vi "Drive Mode.vi"   [LabVIEW 2016]
uses:
  <vilib>/Rock Robotics/WPI/Camera/WPI_CameraExposure Values.ctl
  <vilib>/Rock Robotics/Network Tables/NT Write Boolean.vi
types:
  T1 = typedef "WPI_CameraExposure Values.ctl" = enum16{"Auto", "Flicker-free 50 Hz", "Flicker-free 60 Hz", "Hold current", "Custom"}
  T2 = typedef "WPI_CameraDevRef.ctl" = cluster{"Camera Address":string, "CameraStatus":errorcluster}
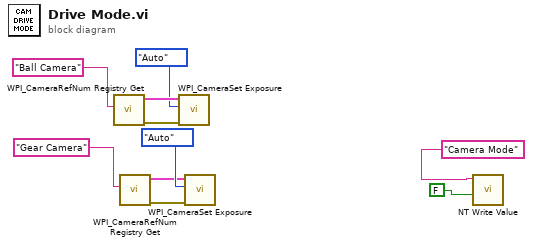
[diagram p0: block diagram]
diagram:
  n1 = call <vilib>:"WPI_CameraRefNum Registry Get.vi"("refnum name"="Ball Camera") -> ("error out"=w4:errorcluster, "CameraDevRef"=w3:T2)  [unwired: 9 in]
  n2 = call <vilib>:"WPI_CameraRefNum Registry Get.vi"("refnum name"="Gear Camera") -> ("error out"=w7:errorcluster, "CameraDevRef"=w8:T2)  [unwired: 9 in]
  n3 = call <vilib>:"WPI_CameraSet Exposure.vi"("error in (no error)"=w4, "Exposure"=WPI_CameraExposure_Values."Auto", "CameraDevRef"=w3) -> ()  [unwired: 1 in, 8 out]
  n4 = call <vilib>:"WPI_CameraSet Exposure.vi"("error in (no error)"=w7, "Exposure"=WPI_CameraExposure_Values."Auto", "CameraDevRef"=w8) -> ()  [unwired: 1 in, 8 out]
  n5 = call-poly <vilib>:"NT Write Value.vi"("Boolean"=FALSE, "Name"="Camera Mode") -> ()  [unwired: 9 in, 1 out]
